vi "mod_Create Gaussian CCDF Trace.vi"(5 "maximum bin (dB)":dbl=0.1 format="%.2f", 9 "bin size (dB)":dbl format="%.2f", 11 "error in (no error)":errorcluster) -> (8 "Gaussian CCDF measurement trace (%)":cluster{"x0":dbl, "dx":dbl, "y":dbl[]} {"y" min=0.0 max=127.0 format="%.2f"; "dx" format="%^.2e"; "x0" format="%^.2e"}, 15 "error out":errorcluster)   [LabVIEW 2020, in "niAMT.lvlib"]
doc: "(c) Copyright 2006, National Instruments, Inc. This VI may not be duplicated, sold, or distributed without written consent from National Instruments."
uses:
  <vilib>/addons/Modulation/niAMT.lvlib
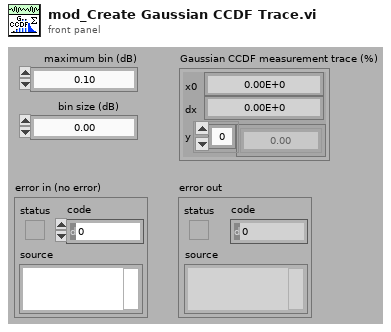
[diagram p1: front panel]
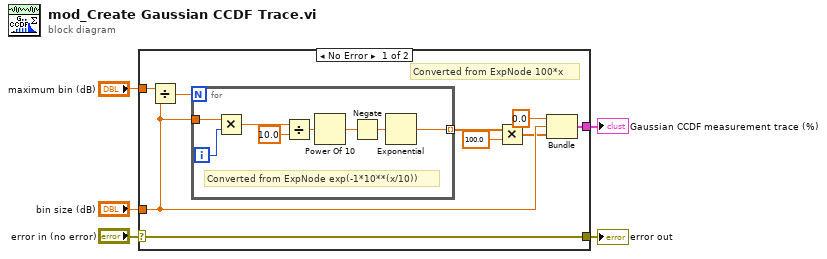
[diagram p0: block diagram]
diagram:
  n1 = case shown="No Error" "error in (no error)" {
    selector: "error in (no error)" -> [w9 w23]
    tunnel: "maximum bin (dB)" -> [w14 _]
    tunnel: "bin size (dB)" -> [w12 _]
    tunnel: [w10 _] -> w3
    tunnel: [w9 w23] -> w1
    frame No Error {
      # "Converted from ExpNode 100*x"
      n2 = Divide(x=w14, y=w12) -> (x/y=w13:dbl)
      n3 = for {
        N: w13 -> [_]
        tunnel: w12 -> [w21]
        tunnel: [w15] -> w7 mode=indexing
        i -> [w22]
        # "Converted from ExpNode exp(-1*10**(x/10))"
        n4 = Multiply(x=w21, y=w22) -> (x*y=w16:dbl)
        n5 = Divide(x=w16, y=10.0) -> (x/y=w18:dbl)
        n6 = Power Of 10(x=w18) -> (10^x=w19:dbl)
        n7 = Negate(x=w19) -> (-x=w20:dbl)
        n8 = Exponential(1:w20) -> (0:w15:dbl)
      }
      n9 = Multiply(x=w7, y=100.0) -> (x*y=w6:dbl[])
      n10 = Bundle(0.0, "bin size (dB)"=w12, w6) -> (w10:cluster{dbl, "bin size (dB)":dbl, dbl[]})  [unwired: 1 out]
    }
    frame Error {
    }
  }
  "Gaussian CCDF measurement trace (%)" <- w3
  "error out" <- w1
